vi "Check Status No Objects.vi"(8 "error in (no error)":errorcluster, 11 "Power Meter in":refnum<class "Power Meter.lvclass">) -> (0 "error out":errorcluster, 1 "Status":string, 2 "Ready?":bool)   [LabVIEW 2009]
doc: "(Dynamic) Check if the instrument is powered on and update its member fields with the instrument's current status. Optionally return a text status message."
uses:
  Power Meter.lvclass
panel:
  out "Cluster 2":T1={"Wavelength"=0.0, "AVG"=0, "Range"=0, "Backlight"=0, "Beeper"=0, "Zero"=0, "Local Lockout"=0, "ATTN"=0, "Run/Stop"=0, "Units"=0, "Averaging Time"=0.0, "Averaging"=TRUE, "Most Recent Power"=0.0, "Filter"=0}
  in  "Cluster":T1={"Wavelength"=0.0, "AVG"=0, "Range"=0, "Backlight"=0, "Beeper"=0, "Zero"=0, "Local Lockout"=0, "ATTN"=0, "Run/Stop"=0, "Units"=0, "Averaging Time"=0.0, "Averaging"=TRUE, "Most Recent Power"=0.0, "Filter"=0}
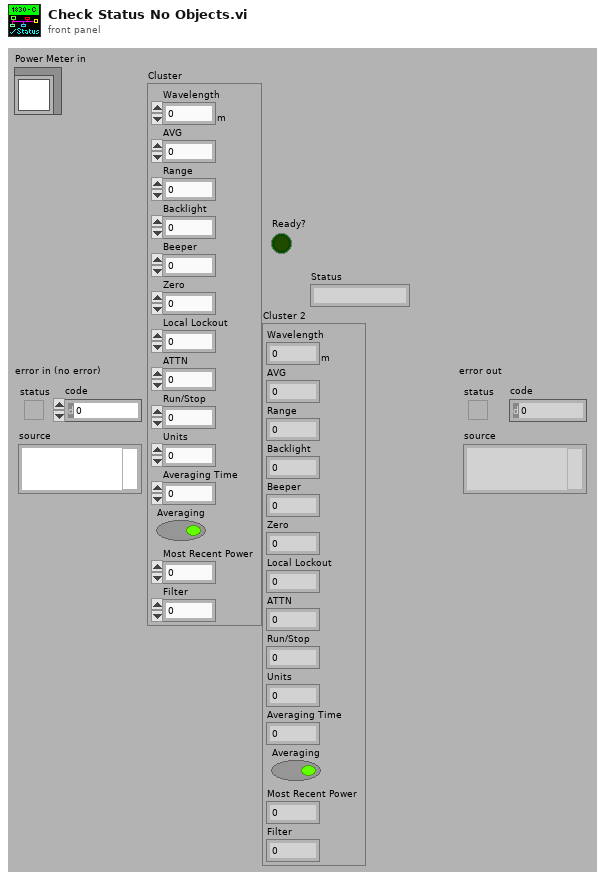
[diagram p1: front panel]
types:
  T1 = cluster{"Wavelength":dbl[unit], "AVG":i32, "Range":i32, "Backlight":i32, "Beeper":i32, "Zero":i32, "Local Lockout":i32, "ATTN":i32, "Run/Stop":i32, "Units":i32, "Averaging Time":dbl, "Averaging":bool, "Most Recent Power":dbl, "Filter":i32}
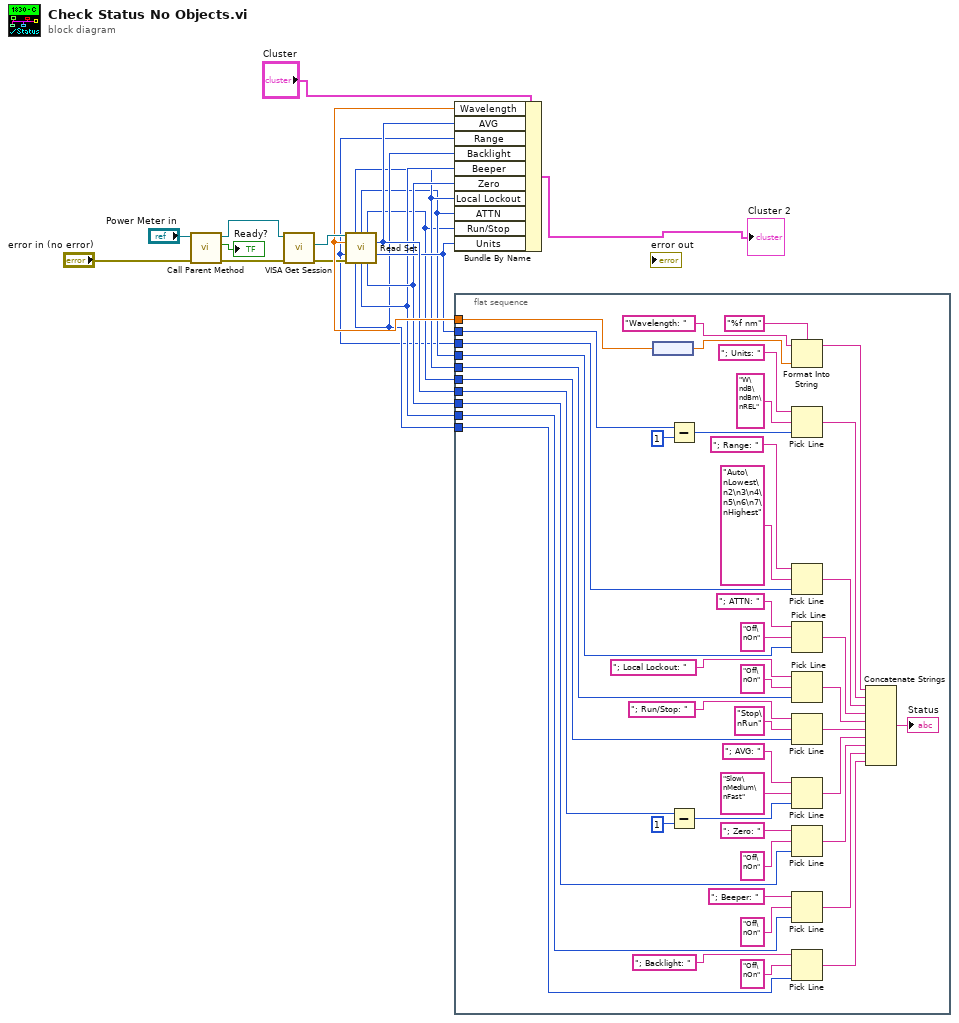
[diagram p0: block diagram]
diagram:
  n1 = call-parent "Call Parent Method"("error in (no error)"="error in (no error)", "Instrument in"="Power Meter in") -> ("error out"=w18:errorcluster, "Ready?"=→"Ready?":bool, "Instrument out"=w19:refnum<class "Power Meter.lvclass">)  [unwired: 6 in, 1 out]
  n2 = call-dynamic "VISA Get Session.vi"("error in (no error)"=w18, "Instrument.lvclass in"=w19) -> ("error out"=w8:errorcluster, "VISA Resource Name"=w16:refnum<visa-resource-name>, "Instrument.lvclass out"=w17:refnum<class "Power Meter.lvclass">)  [unwired: 7 out]
  n3 = call "Read Set.vi"("VISA resource name"=w16, "error in (no error)"=w8) -> ("Local Lockout"=w6:u32, "ATTN"=w5:u32, "Run/Stop"=w4:u32, "VISA resource name out"=w15:refnum<visa-resource-name>, "Wavelength (nnnn)"=w14:dbl[unit], "AVG"=w13:u32, "Range (1:8)"=w3:u32, "Units"=w12:u32, "Backlight"=w9:u32, "Beeper"=w10:u32, "Zero"=w11:u32, "error out"=w7:errorcluster)  [unwired: 2 in]
  n4 = Bundle By Name(cluster="Cluster", "Wavelength"=w14, "AVG"=w13, "Range"=w3, "Backlight"=w9, "Beeper"=w10, "Zero"=w11, "Local Lockout"=w6, "ATTN"=w5, "Run/Stop"=w4, "Units"=w12) -> (→"Cluster 2":T1)
  n5 = flat-sequence {
    tunnel: w12 -> [w60]
    tunnel: w14 -> [w56]
    tunnel: w5 -> [w54]
    tunnel: w3 -> [w50]
    tunnel: w6 -> [w46]
    tunnel: w4 -> [w42]
    tunnel: w13 -> [w38]
    tunnel: w11 -> [w32]
    tunnel: w10 -> [w28]
    tunnel: w9 -> [w24]
    frame #0 {
      n6 = node(w56) -> (w68:dbl)
      n7 = Subtract(x=w60, y=u32 1) -> (x-y=w58:u32)
      n8 = Subtract(x=w38, y=u32 1) -> (x-y=w36:u32)
      n9 = Format Into String(format string="%f nm", initial string="Wavelength: ", w68) -> (resulting string=w63:string)  [unwired: 1 in, 1 out]
      n10 = Pick Line(string ("")="; Units: ", multi-line string="W\ndB\ndBm\nREL", line index=w58) -> (output string=w62:string)
      n11 = Pick Line(string ("")="; Range: ", multi-line string="Auto\nLowest\n2\n3\n4\n5\n6\n7\nHighest", line index=w50) -> (output string=w49:string)
      n12 = Pick Line(string ("")="; ATTN: ", multi-line string="Off\nOn", line index=w54) -> (output string=w53:string)
      n13 = Pick Line(string ("")="; Local Lockout: ", multi-line string="Off\nOn", line index=w46) -> (output string=w45:string)
      n14 = Pick Line(string ("")="; Run/Stop: ", multi-line string="Stop\nRun", line index=w42) -> (output string=w41:string)
      n15 = Pick Line(string ("")="; AVG: ", multi-line string="Slow\nMedium\nFast", line index=w36) -> (output string=w35:string)
      n16 = Pick Line(string ("")="; Zero: ", multi-line string="Off\nOn", line index=w32) -> (output string=w31:string)
      n17 = Pick Line(string ("")="; Beeper: ", multi-line string="Off\nOn", line index=w28) -> (output string=w27:string)
      n18 = Pick Line(string ("")="; Backlight: ", multi-line string="Off\nOn", line index=w24) -> (output string=w23:string)
      n19 = Concatenate Strings(w63, w62, w49, w53, w45, w41, w35, w31, w27, w23) -> (→"Status":string)
    }
  }
